vi "SetLogFormatter.vi"(8 "Error in (no error)":errorcluster, 10 "LogFormatterInterface in":refnum<class "LogFormatterInterface.lvclass">, 11 "LogWriterDb in":refnum<class "LogWriterDb.lvclass">) -> (0 "Error out":errorcluster, 3 "LogWriterDb out":refnum<class "LogWriterDb.lvclass">)   [LabVIEW 2011, in "LogWriterDb.lvclass"]
uses:
  LogWriterDb.lvclass
  Formatter/LogFormatterInterface/LogFormatterInterface.lvclass
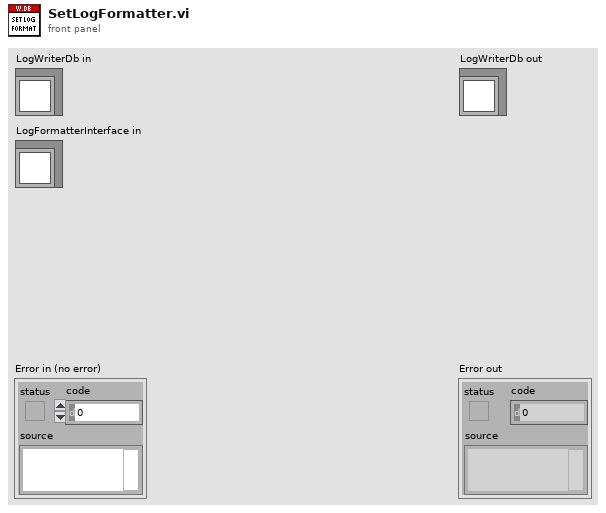
[diagram p1: front panel]
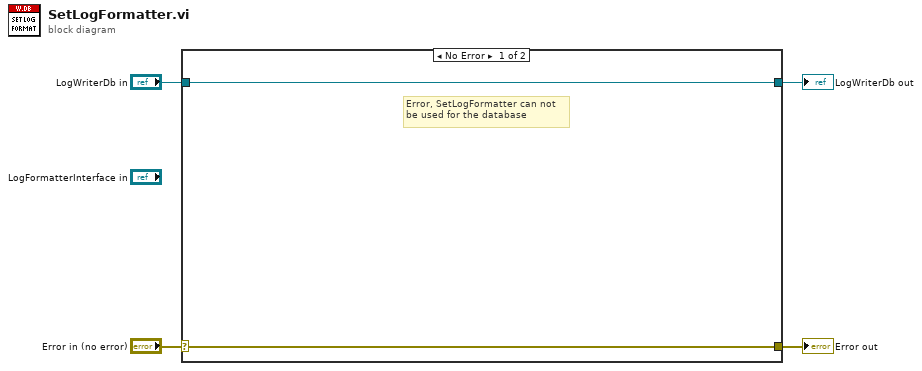
[diagram p0: block diagram]
diagram:
  n1 = case shown="No Error" "Error in (no error)" {
    selector: "Error in (no error)" -> [w5 w8]
    tunnel: [w5 w8] -> w3
    tunnel: [w6 w7] -> w1
    tunnel: "LogWriterDb in" -> [w6 w7]
    frame No Error {
      # "Error, SetLogFormatter can not\nbe used for the database"
    }
    frame Error {
    }
  }
  "Error out" <- w3
  "LogWriterDb out" <- w1
